vi "RSZVB Get Generator Port Resolution Bandwidth.vi"(7 "Generator Port (1)":i32=1, 8 "error in (no error)":errorcluster {"code" format="%.0x"}, 10 "Channel (1)":i32=1, 11 "VISA session":refnum<visa-resource-name>) -> (0 "error out":errorcluster {"code" format="%.0x"}, 3 "dup VISA session":refnum<visa-resource-name>, 9 "Resolution Bandwidth (30.0e6 Hz)":dbl=10000.0 min=1.0 max=30000000.0 format="%^.3e")   [LabVIEW 2011]
doc: "Queries the resolution bandwidth of the analyzer for all partial measurements where an external generator <Gen> is used as a source.\n\nRemote-control command(s):\n[SENSe<Ch>:]BANDwidth|BWIDth[:RESolution]:GENerator<Gen>?"
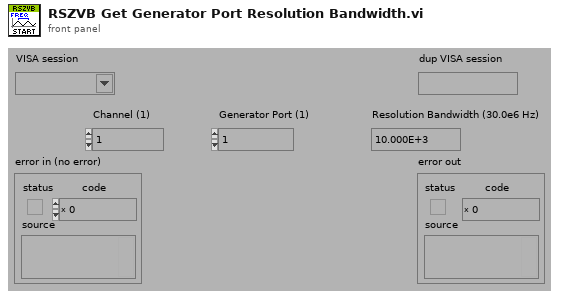
[diagram p1: front panel]
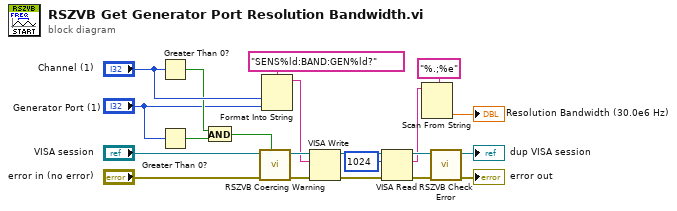
[diagram p0: block diagram]
diagram:
  n1 = Greater Than 0?(x="Channel (1)") -> (x > 0?=w11:bool)
  n2 = Greater Than 0?(x="Generator Port (1)") -> (x > 0?=w12:bool)
  n3 = And(x=w11, y=w12) -> (x .and. y?=w9:bool)
  n4 = call "RSZVB Coercing Warning.vi"("In Range?"=w9, "error in (no error)"="error in (no error)", "VISA session"="VISA session") -> ("error out"=w19:errorcluster, "dup VISA session"=w20:refnum<visa-resource-name>)  [unwired: 7 in]
  n5 = Format Into String(format string="SENS%ld:BAND:GEN%ld?", "Channel (1)", "Generator Port (1)") -> (resulting string=w18:string)  [unwired: 2 in, 1 out]
  n6 = VISA Write(VISA resource name=w20, write buffer=w18, error in (no error)=w19) -> (VISA resource name out=w7:refnum<visa-resource-name>, error out=w8:errorcluster)  [unwired: 1 out]
  n7 = VISA Read(VISA resource name=w7, byte count=u32 1024, error in (no error)=w8) -> (VISA resource name out=w5:refnum<visa-resource-name>, read buffer=w2:string, error out=w6:errorcluster)  [unwired: 1 out]
  n8 = Scan From String(format string="%.;%e", input string=w2) -> (output 1=→"Resolution Bandwidth (30.0e6 Hz)":dbl)  [unwired: 3 in, 3 out]
  n9 = call "RSZVB Check Error.vi"("error in (no error)"=w6, "VISA session"=w5) -> ("error out"=→"error out":errorcluster, "dup VISA session"=→"dup VISA session":refnum<visa-resource-name>)  [unwired: 8 in]
